vi "picoquant_start_stream.vi"(8 "error in (no error)":errorcluster, 11 "hydraharp in":refnum<class "hydraharp.lvclass">) -> (0 "error out":errorcluster, 3 "hydraharp out":refnum<class "hydraharp.lvclass">)   [LabVIEW 2015, in "hydraharp.lvclass"]
uses:
  hydraharp.lvclass
  hydraharp.lvclass/hydraharp.ctl
  hhlib.dll
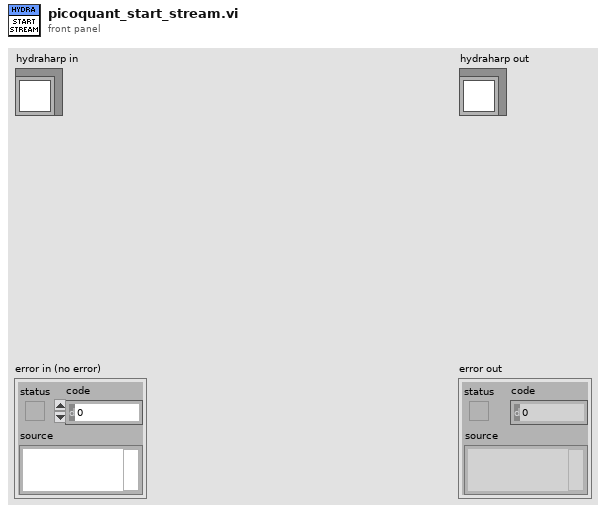
[diagram p1: front panel]
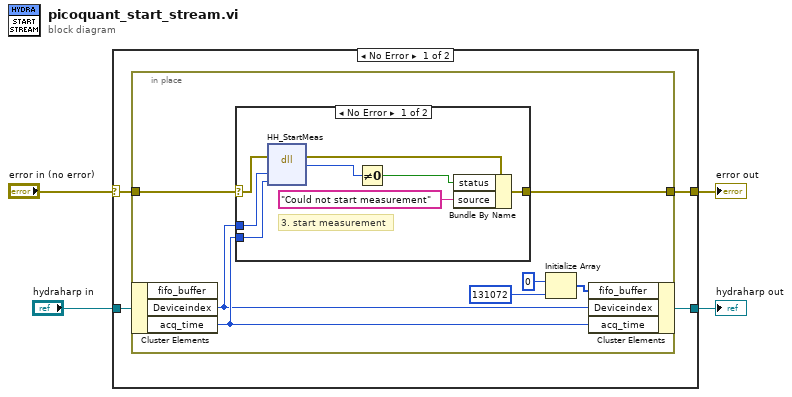
[diagram p0: block diagram]
diagram:
  n1 = case shown="No Error" "error in (no error)" {
    selector: "error in (no error)" -> [w7 w26]
    tunnel: [w5 w26] -> w1
    tunnel: [w6 w25] -> w2
    tunnel: "hydraharp in" -> [w8 w25]
    frame No Error {
      n2 = in-place {
        in-place-border: w7 -> [w9]
        in-place-border: [w11] -> w5
        n3 = in-place-cluster #1(w8) -> ("Deviceindex"=w10:i32, "acq_time"=w12:i32)  [unwired: 1 out]
        n4 = case shown="No Error" w9 {
          selector: w9 -> [w16 w24]
          tunnel: w12 -> [w23 _]
          tunnel: [w18 w24] -> w11
          tunnel: w10 -> [w17 _]
          frame No Error {
            # "3. start measurement"
            n5 = dll-call lib="hhlib.dll" fn="HH_StartMeas"(error in=w16, "devidx"=w17, "tacq"=w23) -> (error out=w21:errorcluster, w22:i32)  [unwired: 4 in, 1 out]
            n6 = Not Equal To 0?(x=w22) -> (x != 0?=w20:bool)
            n7 = Bundle By Name(cluster=w21, "status"=w20, "source"="Could not start measurement") -> (w18:errorcluster)
          }
          frame Error {
          }
        }
        n8 = Initialize Array(u32 0 ("element"), 131072 ("dimension size")) -> (w15:u32[])
        n9 = in-place-cluster #1("fifo_buffer"=w15, "Deviceindex"=w10, "acq_time"=w12) -> (w6:refnum<class "hydraharp.lvclass">)
      }
    }
    frame Error {
    }
  }
  "error out" <- w1
  "hydraharp out" <- w2
